vi "Core Stream Controller.vi"(0 "input valid":bool, 1 "reset":bool, 2 "end continuous mode":bool, 5 "start trigger":bool, 7 "abort":bool, 9 "burst size":u32, 11 "current time":u64, 12 "samples per cycle":u32=1, 13 "future trigger":bool) -> (4 "stream":bool, 6 "state":T1, 8 "samples processed":u32, 10 "stream start time":u64)   [LabVIEW 2025]
uses:
  Stream Control State.ctl
  Stream Control Parameters.ctl
  <instrlib>/_niInstr/Basic Elements/v1/FPGA/niInstr Basic Elements v1 FPGA.lvlib
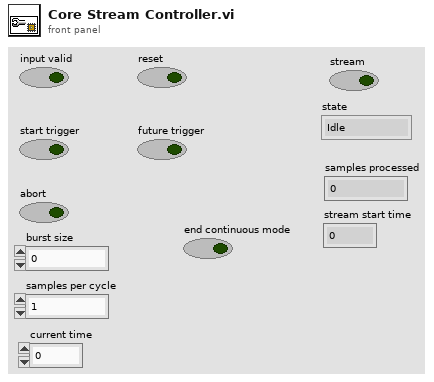
[diagram p1: front panel]
types:
  T1 = typedef "Stream Control State.ctl" = enum16{"Idle", "Active", "WaitForTrigger"}
  T2 = typedef "Stream Control Parameters.ctl" = cluster{"finite":bool, "samples remaining":u32, "state":T1, "samples processed":u32}
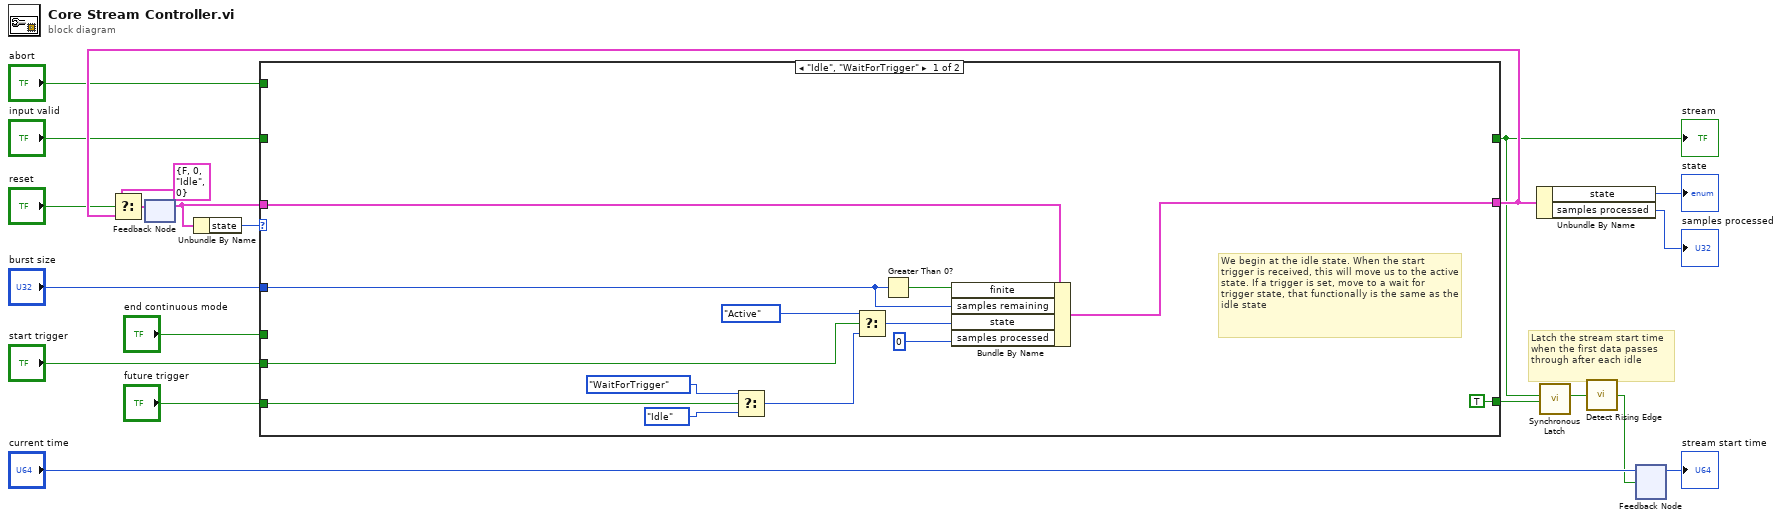
[diagram p0: block diagram]
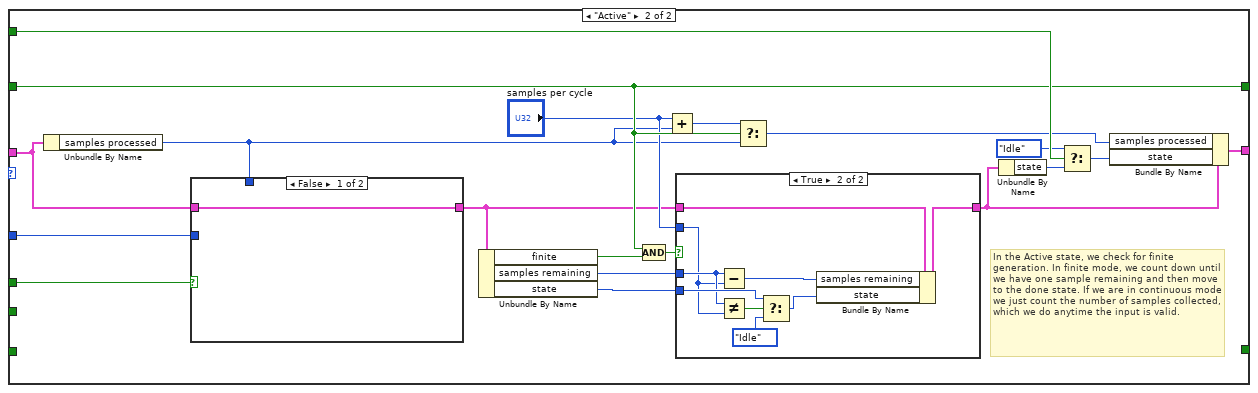
[diagram p2: hidden frame]
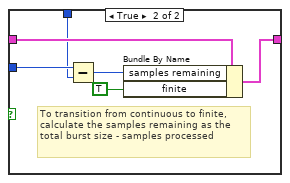
[diagram p3: hidden frame]
diagram:
  # "Latch the stream start time when the first data passes through after each idle"
  n1 = feedback #1() -> (w17:T2)  [unwired: 1 in]
  n2 = Unbundle By Name(w17) -> ("state"=w18:T1)
  n3 = case shown="\"Idle\", \"WaitForTrigger\"" w18 {
    tunnel: "input valid" -> [_ w42]
    tunnel: w17 -> [w29 w36]
    tunnel: "burst size" -> [w32 w34]
    tunnel: [w22 w45] -> w19
    tunnel: [_ w42] -> w5
    tunnel: "start trigger" -> [w24 _]
    tunnel: "abort" -> [_ w44]
    tunnel: "end continuous mode" -> [_ w38]
    tunnel: [TRUE _] -> w4
    tunnel: "future trigger" -> [w23 _]
    frame "Idle", "WaitForTrigger" {
      # "We begin at the idle state. When the start trigger is received, this will move us to the active state. If a trigger is set, move to a wait for trigger state, that functionally is the same as the idle state"
      n4 = Select(t=Stream_Control_State."WaitForTrigger", s=w23, f=Stream_Control_State."Idle" ("t")) -> (s? t:f=w25:T1)
      n5 = Select(t=Stream_Control_State."Active", s=w24, f=w25) -> (s? t:f=w30:T1)
      n6 = Greater Than 0?(x=w32) -> (x > 0?=w33:bool)
      n7 = Bundle By Name(cluster=w29, "finite"=w33, "samples remaining"=w32, "state"=w30, "samples processed"=u32 0) -> (w22:T2)
    }
    frame "Active" {
      # "In the Active state, we check for finite generation. In finite mode, we count down until we have one sample remaining and then move to the done state. If we are in continuous mode we just count the number of samples collected, which we do anytime the input is valid."
      n8 = Unbundle By Name(w36) -> ("samples processed"=w35:u32)
      n9 = case shown="False" w38 {
        tunnel: w36 -> [w53 w59]
        tunnel: [w53 w57] -> w37
        tunnel: w35 -> [_ w55]
        tunnel: w34 -> [_ w56]
        frame False {
        }
        frame True {
          # "To transition from continuous to finite, calculate the samples remaining as the total burst size - samples processed"
          n10 = Subtract(x=w56, y=w55) -> (x-y=w54:u32)
          n11 = Bundle By Name(cluster=w59, "samples remaining"=w54, "finite"=TRUE) -> (w57:T2)
        }
      }
      n12 = Unbundle By Name(w37) -> ("finite"=w51:bool, "samples remaining"=w52:u32, "state"=w49:T1)
      n13 = Compound Arithmetic op=AND(w42, w51) -> (w50:bool)
      n14 = Add(x="samples per cycle", y=w35) -> (x+y=w40:u32)
      n15 = case shown="True" w50 {
        tunnel: [w60 w69] -> w46
        tunnel: w37 -> [w60 w68]
        tunnel: w52 -> [_ w63]
        tunnel: w49 -> [_ w65]
        tunnel: "samples per cycle" -> [_ w61]
        frame False {
        }
        frame True {
          n16 = Subtract(x=w63, y=w61) -> (x-y=w62:u32)
          n17 = Not Equal?(x=w63, y=w61) -> (x != y?=w67:bool)
          n18 = Select(t=w65, s=w67, f=Stream_Control_State."Idle" ("state")) -> (s? t:f=w66:T1)
          n19 = Bundle By Name(cluster=w68, "samples remaining"=w62, "state"=w66) -> (w69:T2)
        }
      }
      n20 = Select(t=w40, s=w42, f=w35) -> (s? t:f=w41:u32)
      n21 = Unbundle By Name(w46) -> ("state"=w48:T1)
      n22 = Select(t=Stream_Control_State."Idle", s=w44, f=w48) -> (s? t:f=w47:T1)
      n23 = Bundle By Name(cluster=w46, "samples processed"=w41, "state"=w47) -> (w45:T2)
    }
  }
  "stream" <- w5
  n24 = Select(t=T2 {"finite"=FALSE, "samples remaining"=0, "state"=enum."Idle", "samples processed"=0} ("Cluster"), s="reset", f=w19) -> (s? t:f=w16:T2)
  n25 = feedback-in #1(w16) -> ()
  n26 = Unbundle By Name(w19) -> ("state"=→"state":T1, "samples processed"=→"samples processed":u32)
  n27 = call <instrlib>:"Synchronous Latch.vi"("clear"=w4, "set"=w5) -> ("out"=w3:bool)  [unwired: 9 in]
  n28 = call <instrlib>:"Detect Rising Edge.vi"("signal"=w3) -> ("edge detected"=w2:bool)  [unwired: 14 in]
  n29 = feedback-in #2("current time", w2) -> ()
  n30 = feedback #2() -> (→"stream start time":u64)  [unwired: 1 in]
